vi "Configure Measurement (Harmonic).vi"(0 "VISA resource name":refnum<visa-resource-name>, 1 "Auto Fundamental Frequency (T: Enable)":bool=TRUE, 2 "Manual Fundamental Frequency  (1E+7 Hz)":dbl=10000000.0, 5 "Frequency Step  (1E+9 Hz)":dbl=1000000000.0, 11 "error in (no error)":errorcluster, 12 "Auto Dwell Time (T: Enable)":bool=TRUE, 13 "Dwell Time (1 s)":dbl=1.0) -> (4 "VISA resource name out":refnum<visa-resource-name>, 15 "error out":errorcluster)   [LabVIEW 2014, in "Agilent MXA Series.lvlib"]
doc: "Sets the harmonic measurement parameters."
uses:
  Agilent MXA Series.lvlib
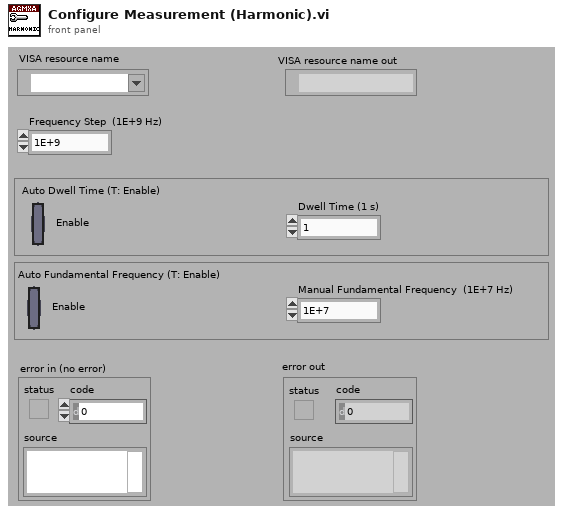
[diagram p1: front panel]
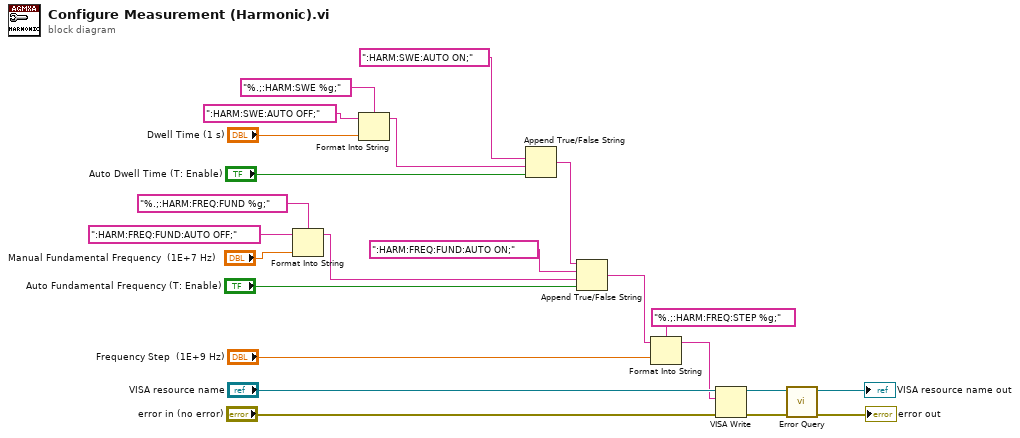
[diagram p0: block diagram]
diagram:
  n1 = Format Into String(format string="%.;:HARM:FREQ:FUND %g;", initial string=":HARM:FREQ:FUND:AUTO OFF;", "Manual Fundamental Frequency  (1E+7 Hz)") -> (resulting string=w14:string)  [unwired: 1 in, 1 out]
  n2 = Format Into String(format string="%.;:HARM:SWE %g;", initial string=":HARM:SWE:AUTO OFF;", "Dwell Time (1 s)") -> (resulting string=w7:string)  [unwired: 1 in, 1 out]
  n3 = Append True/False String(1:"Auto Dwell Time (T: Enable)", 2:w7, 3:":HARM:SWE:AUTO ON;" ("true string")) -> (0:w5:string)  [unwired: 1 in]
  n4 = Append True/False String(1:"Auto Fundamental Frequency (T: Enable)", 2:w14, 3:":HARM:FREQ:FUND:AUTO ON;" ("true string"), 4:w5) -> (0:w3:string)
  n5 = Format Into String(format string="%.;:HARM:FREQ:STEP %g;", initial string=w3, "Frequency Step  (1E+9 Hz)") -> (resulting string=w1:string)  [unwired: 1 in, 1 out]
  n6 = VISA Write(VISA resource name="VISA resource name", write buffer=w1, error in (no error)="error in (no error)") -> (VISA resource name out=w20:refnum<visa-resource-name>, error out=w21:errorcluster)  [unwired: 1 out]
  n7 = call "Error Query.vi"("error in (no error)"=w21, "VISA resource name"=w20) -> ("error out"=→"error out":errorcluster, "VISA resource name out"=→"VISA resource name out":refnum<visa-resource-name>)  [unwired: 6 in, 2 out]
